vi "MeasurementConfigGlobals.vi"() -> ()   [LabVIEW 2019]
panel:
  in  "Array":T1(array[cluster])
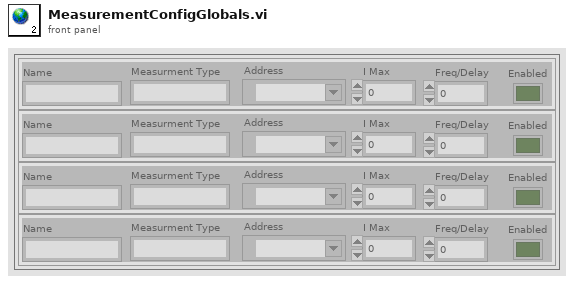
[diagram p1: front panel]
types:
  T1 = cluster{"Name":string, "Measurment Type":string, "I Max":dbl, "Freq/Delay":dbl, "Address":refnum<visa-resource-name>, "Enabled":bool}[]
diagram:
